vi "Run Stream VI.vi"(8 "error in (no error)":errorcluster, 11 "Filter_Wheel in":refnum<class "Filter_Wheel.lvclass">) -> (0 "error out":errorcluster, 3 "Filter_Wheel out":refnum<class "Filter_Wheel.lvclass">)   [LabVIEW 2018, in "Filter_Wheel.lvclass"]
uses:
  Filter_Wheel.lvclass
  Filter_Wheel.lvclass/Filter_Wheel.ctl
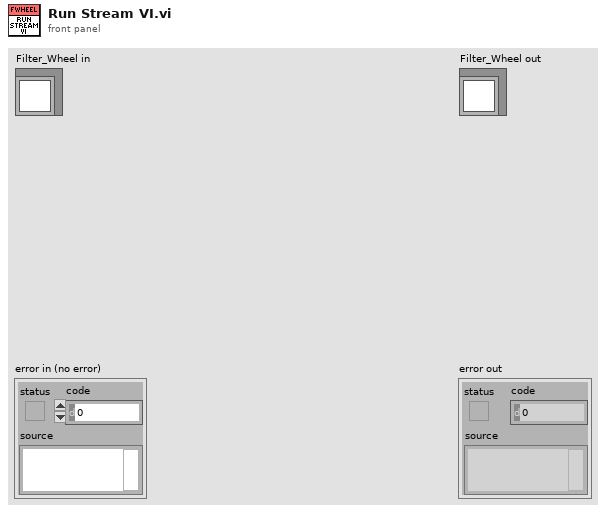
[diagram p1: front panel]
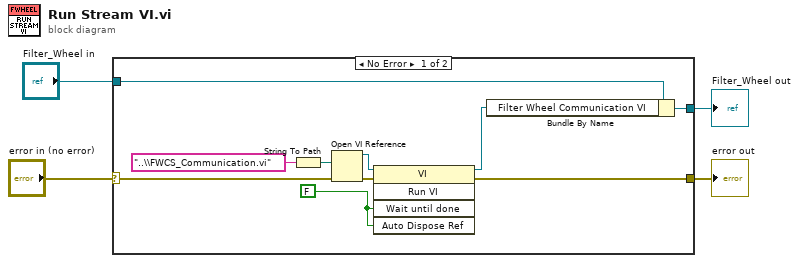
[diagram p0: block diagram]
diagram:
  n1 = case shown="No Error" "error in (no error)" {
    selector: "error in (no error)" -> [w14 w16]
    tunnel: [w12 w16] -> w3
    tunnel: [w8 w15] -> w1
    tunnel: "Filter_Wheel in" -> [w9 w15]
    frame No Error {
      w5 = FALSE ("Wait Until Done")
      n2 = String To Path(string="..\\FWCS_Communication.vi") -> (path=w10:path)
      n3 = Open VI Reference(vi path=w10, error in (no error)=w14) -> (vi reference=w6:refnum<vi>, error out=w13:errorcluster)  [unwired: 4 in]
      n4 = invoke class="VI" method="Run VI"(reference=w6, error in=w13, "Wait until done"=w5, "Auto Dispose Ref"=w5) -> (reference out=w7:refnum<vi>, error out=w12:errorcluster)  [unwired: 1 in, 3 out]
      n5 = Bundle By Name(cluster=w9, "Filter Wheel Communication VI"=w7) -> (w8:refnum<class "Filter_Wheel.lvclass">)
    }
    frame Error {
    }
  }
  "error out" <- w3
  "Filter_Wheel out" <- w1
